vi "sub_GetVIImages.vi"(2 "Save screenshot dir":path, 3 "Selected VI":path) -> (0 "Block Diagram":picture, 1 "Front Panel":picture)   [LabVIEW 2012]
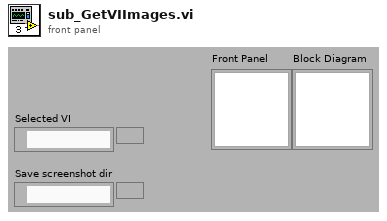
[diagram p1: front panel]
types:
  T1 = typedef "imagedata.ctl" = cluster{"image type":i32, "image depth":i32, "image":u8[], "mask":u8[], "colors":u32[], "Rectangle":cluster{"left":i16, "top":i16, "right":i16, "bottom":i16}}
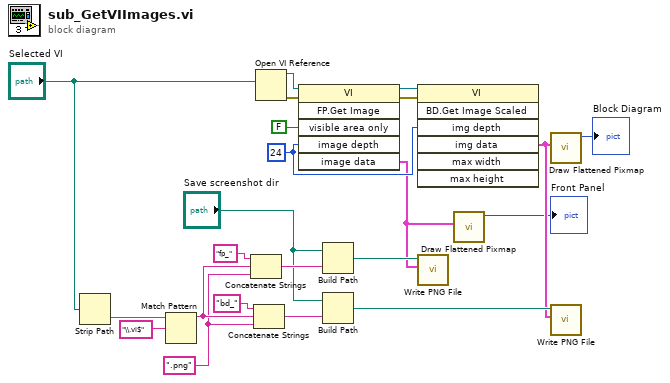
[diagram p0: block diagram]
diagram:
  w7 = ".png" ("string")
  w19 = 24 ("image depth")
  n1 = Strip Path(path="Selected VI") -> (name=w17:string)  [unwired: 1 out]
  n2 = Match Pattern(string=w17, regular expression="\\.vi$") -> (before substring=w16:string)  [unwired: 1 in, 3 out]
  n3 = Concatenate Strings("fp_" ("string"), w16, w7) -> (w14:string)
  n4 = Concatenate Strings("bd_" ("string"), w16, w7) -> (w15:string)
  n5 = Open VI Reference(vi path="Selected VI") -> (vi reference=w21:refnum<vi>, error out=w10:errorcluster)  [unwired: 5 in]
  n6 = invoke class="VI" method="FP.Get Image"(reference=w21, error in=w10, "visible area only"=FALSE ("Visible Area Only"), "image depth"=w19) -> (reference out=w20:refnum<vi>, error out=w11:errorcluster, "image data"=w3:T1)  [unwired: 2 in, 3 out]
  n7 = Build Path(base path="Save screenshot dir", name or relative path=w14) -> (appended path=w13:path)
  n8 = Build Path(base path="Save screenshot dir", name or relative path=w15) -> (appended path=w12:path)
  n9 = invoke class="VI" method="BD.Get Image Scaled"(reference=w20, error in=w11, "img depth"=w19) -> ("img data"=w4:T1)  [unwired: 4 in, 6 out]
  n10 = call <vilib>:"Write PNG File.vi"("image data"=w3, "path to PNG file"=w13) -> ()  [unwired: 8 in, 2 out]
  n11 = call <vilib>:"Draw Flattened Pixmap.vi"("image data"=w3) -> ("new picture"=→"Front Panel":picture)  [unwired: 8 in]
  n12 = call <vilib>:"Draw Flattened Pixmap.vi"("image data"=w4) -> ("new picture"=→"Block Diagram":picture)  [unwired: 8 in]
  n13 = call <vilib>:"Write PNG File.vi"("image data"=w4, "path to PNG file"=w12) -> ()  [unwired: 8 in, 2 out]
